vi "Update AO Sweep Status All False.vi"(8 "error in (no error)":errorcluster, 11 "Generator in":refnum<class "Generator.lvclass">) -> (0 "error out":errorcluster, 3 "Generator out":refnum<class "Generator.lvclass">)   [LabVIEW 2019, in "Generator.lvclass"]
uses:
  Generator.lvclass
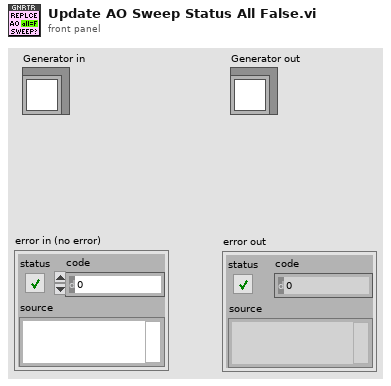
[diagram p1: front panel]
types:
  T1 = typedef "Generator.lvclass/AO.Channel--Cluster--Array.ctl" = T2[]
  T2 = typedef "Generator.lvclass/AO.Channel--Cluster.ctl" = cluster{"Enable?":bool, "Channel":i32, "Amplitude":dbl, "Offset":dbl, "Frequency":dbl, "Phase":dbl, "Function":T3, "Sweeping?":bool, "Limit AC?":bool, "Limit DC?":bool, "Duty Cycle?":bool, "Duty Cycle":dbl}
  T3 = typedef "Generator.lvclass/AO.Channel.Function--Enum.ctl" = enum16{"sine", "square", "triangle", "saw"}
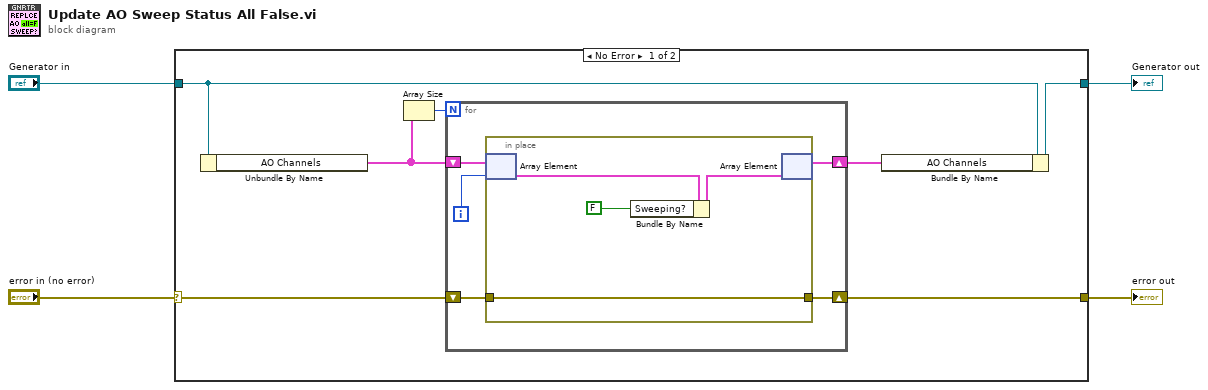
[diagram p0: block diagram]
diagram:
  n1 = case shown="No Error" "error in (no error)" {
    selector: "error in (no error)" -> [w10 w22]
    tunnel: "Generator in" -> [w11 w21]
    tunnel: [w8 w22] -> w2
    tunnel: [w7 w21] -> w1
    frame No Error {
      n2 = Unbundle By Name(w11) -> ("AO Channels"=w5:T1)
      n3 = Array Size(array=w5) -> (size(s)=w6:i32)
      n4 = for {
        N: w6 -> [_]
        shift-right: [w15] -> w8
        shift-left: w10 -> [w16]
        shift-right: [w12] -> w9
        shift-left: w5 -> [w14]
        i -> [w13]
        n5 = in-place {
          in-place-border: w16 -> [w19]
          in-place-border: [w19] -> w15
          n6 = in-place-array #1(w14, w13) -> (w18:T2)
          n7 = Bundle By Name(cluster=w18, "Sweeping?"=FALSE) -> (w17:T2)
          n8 = in-place-array #1(w17) -> (w12:T1)  [unwired: 1 out]
        }
      }
      n9 = Bundle By Name(cluster=w11, "AO Channels"=w9) -> (w7:refnum<class "Generator.lvclass">)
    }
    frame Error {
    }
  }
  "Generator out" <- w1
  "error out" <- w2
